vi "Disable table edit.vi"() -> ()   [LabVIEW 2015]
uses:
  <vilib>/Utility/cursorutil.llb/Set Cursor (Icon Pict).vi
panel:
  in  "Table Control":string[][](table)
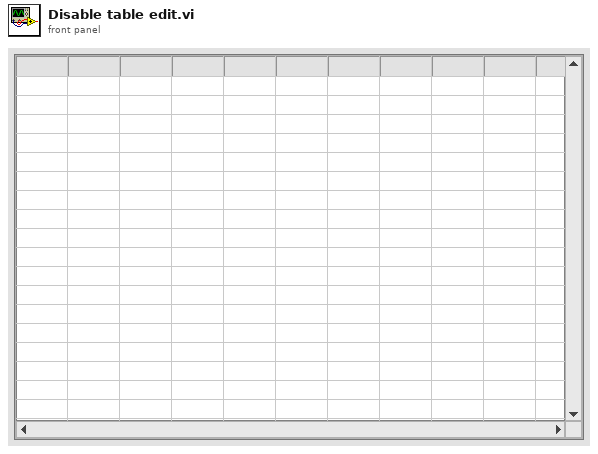
[diagram p1: front panel]
types:
  T1 = typedef "LVPoint32TypeDef.ctl" = cluster{"Horizontal":i32, "Vertical":i32}
  T2 = typedef "LVRowAndColumnTypeDef.ctl" = cluster{"Row":i32, "Column":i32}
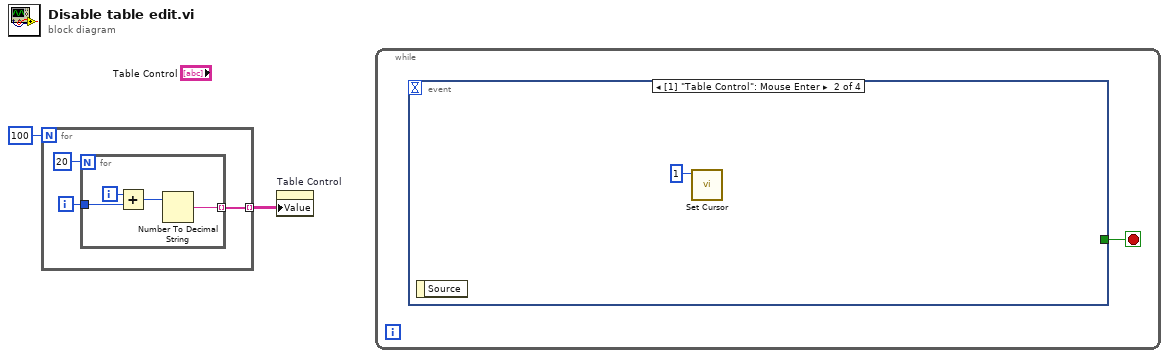
[diagram p0: block diagram]
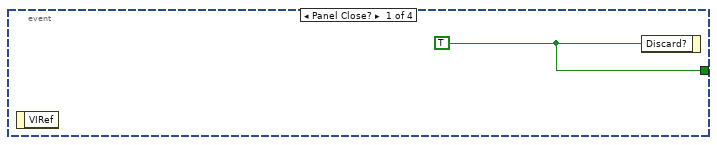
[diagram p2: hidden frame]
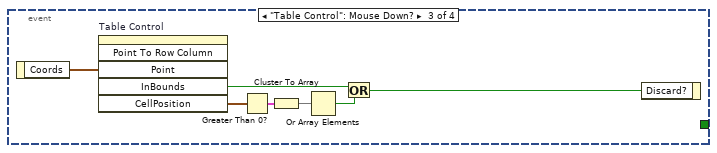
[diagram p3: hidden frame]
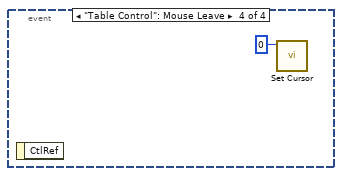
[diagram p4: hidden frame]
diagram:
  n1 = for {
    N: 100 -> [_]
    tunnel: [w5] -> w2 mode=indexing
    i -> [w4]
    n2 = for {
      N: 20 -> [_]
      tunnel: [w9] -> w5 mode=indexing
      tunnel: w4 -> [w7]
      i -> [w8]
      n3 = Add(x=w8, y=w7) -> (x+y=w6:i32)
      n4 = Number To Decimal String(number=w6) -> (decimal integer string=w9:string)  [unwired: 1 in]
    }
  }
  n5 = property on="Table Control" class="Tbl (strict)"("Value"=w2) -> ()  [unwired: 2 in, 2 out]
  n6 = while {
    stop <- w10 stop-if-true
    n7 = event shown="[1] \"Table Control\": Mouse Enter" {
      selector: _ -> [_ _ _ _]
      dyn-events: _ -> [_ _ _ _]
      timeout: _ -> [_ _ _ _]
      tunnel: [w11 _ _ _] -> w10
      event Panel Close? {
        w11 = TRUE
        n8 = event-data() -> ()  [unwired: 1 in, 1 out]
        n9 = event-data("Discard?"=w11) -> ()  [unwired: 1 in, 1 out]
      }
      event "Table Control": Mouse Enter {
        n10 = event-data() -> ()  [unwired: 1 in, 1 out]
        n11 = call-poly <vilib>:"Set Cursor.vi"("icon"=u16 1) -> ()  [unwired: 9 in, 2 out]
      }
      event "Table Control": Mouse Down? {
        n12 = event-data() -> ("Coords"=w19:T1)  [unwired: 1 in]
        n13 = invoke on="Table Control" class="Tbl (strict)" method="Point To Row Column"("Point"=w19) -> ("InBounds"=w14:bool, "CellPosition"=w18:T2)  [unwired: 5 in, 4 out]
        n14 = Greater Than 0?(x=w18) -> (x > 0?=w17:cluster{"Row":bool, "Column":bool})
        n15 = Cluster To Array(cluster=w17) -> (array=w16:bool[])
        n16 = Or Array Elements(Boolean array=w16) -> (logical OR=w15:bool)
        n17 = Or(x=w14, y=w15) -> (x .or. y?=w13:bool)
        n18 = event-data("Discard?"=w13) -> ()  [unwired: 1 in, 1 out]
      }
      event "Table Control": Mouse Leave {
        n19 = event-data() -> ()  [unwired: 1 in, 1 out]
        n20 = call-poly <vilib>:"Set Cursor.vi"("icon"=u16 0) -> ()  [unwired: 9 in, 2 out]
      }
    }
  }
